vi "RUN.vi"() -> ()   [LabVIEW 2011]
panel:
  out "concatenated string":string
  out "Galil Error":errorcluster
  in  "Stop":bool
  in  "Initial Encoder Counts":string="0" caption="Enter number in encoder counts, 0 is middle, -650000 fully entended; 650000 fully retracted"
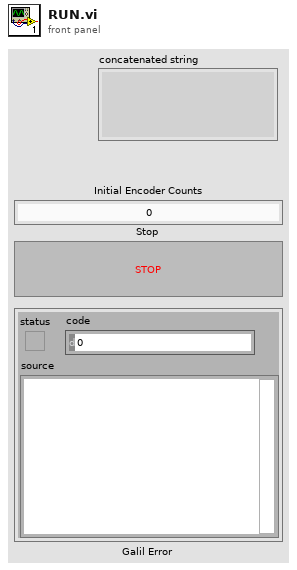
[diagram p1: front panel]
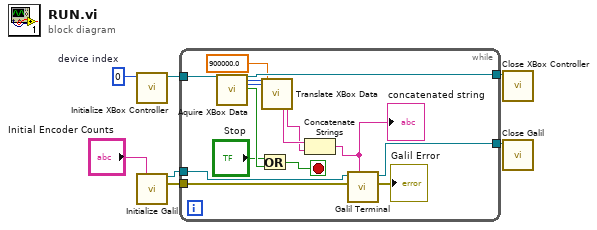
[diagram p0: block diagram]
diagram:
  w2 = 0  # device index
  n1 = call "Initialize XBox Controller.vi"("XBox Device Index"=w2) -> ("Device ID"=w6:refnum<k1>)  [unwired: 8 in, 2 out]
  n2 = call "Initialize Galil.vi"("Initial Encoder Counts"="Initial Encoder Counts") -> ("reference out 3"=w4:refnum<k7>, "error out 3"=w1:errorcluster)  [unwired: 9 in, 4 out]
  n3 = while {
    tunnel: [w22] -> w7
    tunnel: w6 -> [w21]
    tunnel: w4 -> [w16]
    tunnel: [w13] -> w3
    tunnel: w1 -> [w9]
    stop <- w18 stop-if-true
    n4 = call "Aquire XBox Data.vi"("device ID"=w21) -> ("device ID 2"=w22:refnum<k1>, "Steer Axis"=w20:i32, "Drive Axis"=w19:i32, "E-Stop (Button B)"=w17:bool)  [unwired: 19 in, 4 out]
    n5 = Or(x="Stop", y=w17) -> (x .or. y?=w18:bool)
    n6 = call "Translate XBox Data.vi"("Steer Axis"=w20, "Drive Axis"=w19, "Limit Count Range"=900000.0) -> ("Steer Value Output String"=w11:string, "Drive Value Output String"=w10:string)  [unwired: 17 in, 6 out]
    n7 = Concatenate Strings(w11, w10) -> (w15:string)
    "concatenated string" <- w15
    n8 = call "Galil Terminal.vi"("Command Input"=w15, "Galil Error In"=w9, "reference out 2"=w16) -> ("Galil Error Out"=→"Galil Error":errorcluster, "reference out 3"=w13:refnum<k7>)  [unwired: 6 in, 1 out]
  }
  n9 = call "Close XBox Controller.vi"("Device ID In"=w7) -> ()  [unwired: 10 in, 1 out]
  n10 = call "Close Galil.vi"("reference out 2"=w3) -> ()  [unwired: 9 in, 2 out]
